vi "Write Library Member Name Replacement.vi"(10 "Library Member Name Replacement":T1, 11 "ProjectItem in":refnum<class "Search.lvclass">) -> (3 "ProjectItem out":refnum<class "Search.lvclass">)   [LabVIEW 2016, in "Search.lvclass"]
uses:
  Search.lvclass
  Typedefs/LibraryMemberNameReplacement.ctl
  Search.lvclass/Search.ctl
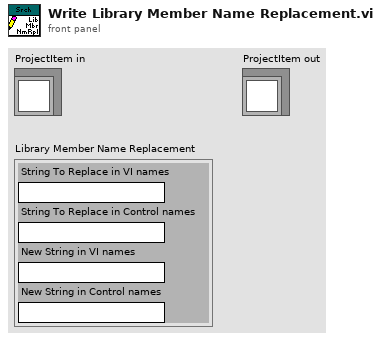
[diagram p1: front panel]
types:
  T1 = typedef "LibraryMemberNameReplacement.ctl" = cluster{"String To Replace in VI names":string, "String To Replace in Control names":string, "New String in VI names":string, "New String in Control names":string}
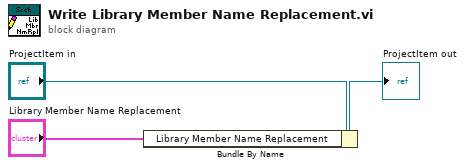
[diagram p0: block diagram]
diagram:
  n1 = Bundle By Name(cluster="ProjectItem in", "Library Member Name Replacement"="Library Member Name Replacement") -> (→"ProjectItem out":refnum<class "Search.lvclass">)
